vi "Impedance tube v0.5.vi"() -> ()   [LabVIEW 2021]
uses:
  <vilib>/ptbypt/Frequency Domain.llb/Real FFT PtByPt.vi
  <vilib>/express/express analysis/Spectral/Block/exnSpectralBlock spectral measurements RMS poly.vi
  <vilib>/express/express analysis/Spectral/Block/exnSpectralBlock spectral measurements RMS DDT.vi
  <vilib>/express/express analysis/Spectral/XNode/ExpressSpectralMeasurementsBlockNode.xnode
  <vilib>/express/express arith-compare/Formula/XNode/ExpressFormulaBlockNode.xnode
  <vilib>/ptbypt/NI_PtbyPt.lvlib
panel:
  out "Reflection Coefficient r":dbl[](graph)
  in  "number of samples":i32=2048
  out "Absorption Coefficient":dbl[](graph)
  out "Waveform Graph 2":dynamicdata(graph)
  out "MIC 2":dynamicdata(graph)
  out "FFT2":dynamicdata(graph)
  out "MIC 2":dbl
  out "FFT1":dynamicdata(graph)
  out "MIC 1":dynamicdata(graph)
  out "MIC 1":dbl
  in  "stop (F)":bool
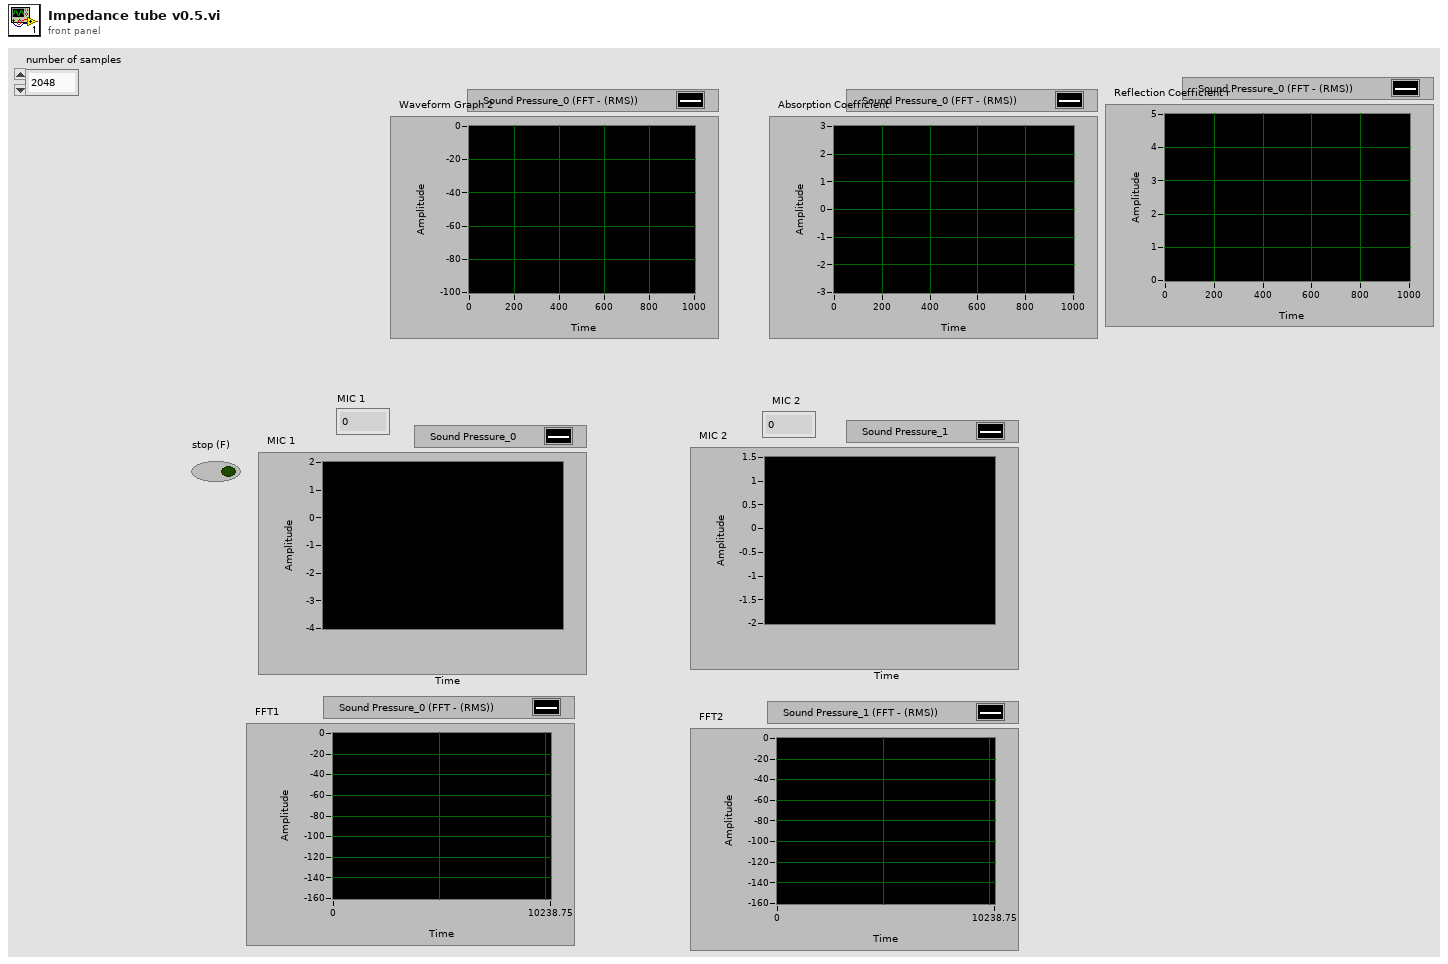
[diagram p1: front panel]
types:
  T1 = cluster{"averaging mode":u16, "weighting mode":u16, "number of averages":u32}
  T2 = cluster{"dB On (F)":bool, "unwrap phase (F)":bool, "convert to degree (F)":bool}
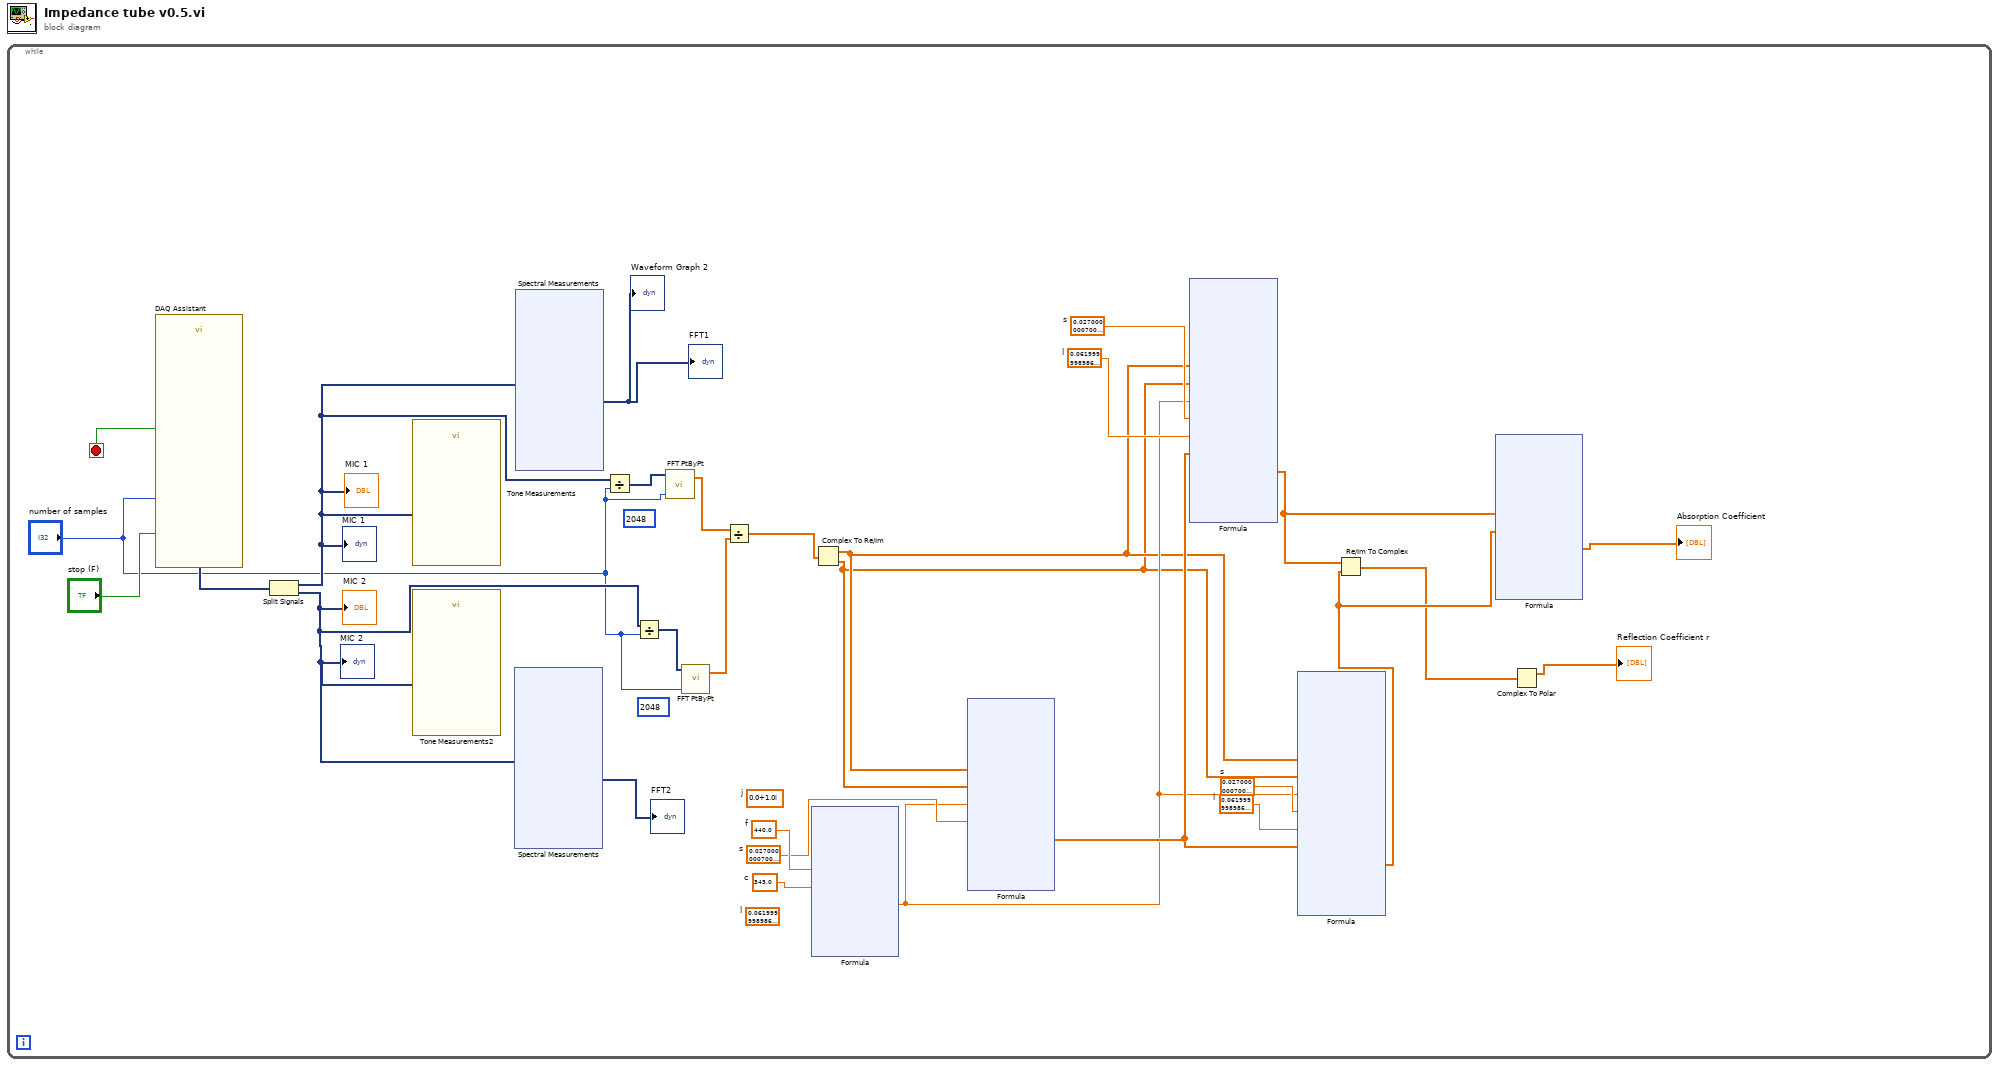
[diagram p0: block diagram]
diagram:
  n1 = while {
    stop <- w28 stop-if-true
    (unwired) 2048 ("number of samples")
    (unwired) 2048 ("number of samples")
    w15 = sgl 0.062  # l
    w16 = sgl 0.027  # s
    w17 = sgl 0.062  # l
    w18 = sgl 0.027  # s
    (unwired) sgl 0.062  # l
    w21 = sgl 440.0  # f
    w19 = sgl 0.027  # s
    w20 = sgl 343.0  # c
    (unwired) csg 0.0+1.0i  # j
    n2 = call "DAQ Assistant"("number of samples"="number of samples", "stop (F)"="stop (F)") -> ("data"=w27:dynamicdata, "stopped"=w28:bool)  [unwired: 14 in, 2 out]
    n3 = Split Signals(w27) -> (w8:dynamicdata, w6:dynamicdata)  [unwired: 2 in]
    "MIC 1" <- w8
    "MIC 1" <- w8
    "MIC 2" <- w6
    "MIC 2" <- w6
    n4 = call "Tone Measurements"("Signals"=w8) -> ()  [unwired: 8 in, 3 out]
    n5 = call "Tone Measurements2"("Signals"=w6) -> ()  [unwired: 8 in, 3 out]
    n6 = xnode "Spectral Measurements"("Signals"=w6) -> ("FFT - (RMS)"=→"FFT2":dynamicdata)  [unwired: 1 in, 2 out]
    n7 = xnode "Spectral Measurements"("Signals"=w8) -> ("FFT - (RMS)"=→"FFT1" →"Waveform Graph 2":dynamicdata)  [unwired: 1 in, 2 out]
    n8 = Divide(x=w8, y="number of samples") -> (x/y=w7:dynamicdata)
    n9 = Divide(x=w6, y="number of samples") -> (x/y=w5:dynamicdata)
    n10 = call-poly <vilib>:"FFT PtByPt.vi"("sample length"="number of samples", "x"=w7) -> ("FFT{X}"=w22:cdb[])  [unwired: 2 in, 1 out]
    n11 = call-poly <vilib>:"FFT PtByPt.vi"("sample length"="number of samples", "x"=w5) -> ("FFT{X}"=w24:cdb[])  [unwired: 2 in, 1 out]
    n12 = Divide(x=w22, y=w24) -> (x/y=w23:cdb[])
    n13 = xnode "Formula"("f"=w21, "c"=w20) -> ("Result"=w13:sgl)  [unwired: 1 in, 1 out]
    n14 = Complex To Re/Im(x + iy=w23) -> (x=w12:dbl[], y=w11:dbl[])
    n15 = xnode "Formula"("Hr"=w12, "Hi"=w11, "k"=w13, "s"=w19) -> ("Result"=w14:dbl[])  [unwired: 1 in, 1 out]
    n16 = xnode "Formula"("Hr"=w12, "Hi"=w11, "k"=w13, "s"=w18, "l"=w17, "D"=w14) -> ("Result"=w3:dbl[])  [unwired: 1 in, 1 out]
    n17 = xnode "Formula"("Hr"=w12, "Hi"=w11, "k"=w13, "s"=w16, "l"=w15, "D"=w14) -> ("Result"=w10:dbl[])  [unwired: 1 in, 1 out]
    n18 = Re/Im To Complex(1:w10, 2:w3) -> (0:w2:cdb[])
    n19 = xnode "Formula"("Rr"=w3, "Ri"=w10) -> ("Result"=→"Absorption Coefficient":dbl[])  [unwired: 1 in, 1 out]
    n20 = Complex To Polar(r * e^(i*theta)=w2) -> (r=→"Reflection Coefficient r":dbl[])  [unwired: 1 out]
  }
